vi "ex_getWaveformName.vi"(8 "error in (no error)":errorcluster, 10 "TimeColumnMode":T1, 11 "Dynamic Data":waveform(dbl)[](array[waveform])) -> (0 "error out":errorcluster, 3 "WaveName":string[](array[string]))   [LabVIEW 2017]
uses:
  <vilib>/express/express shared/NI_ExcelFile/Ctrls/TimeColumnMode.ctl
  <vilib>/express/express shared/NI_ExcelFile/NI_ExcelFile.lvlib
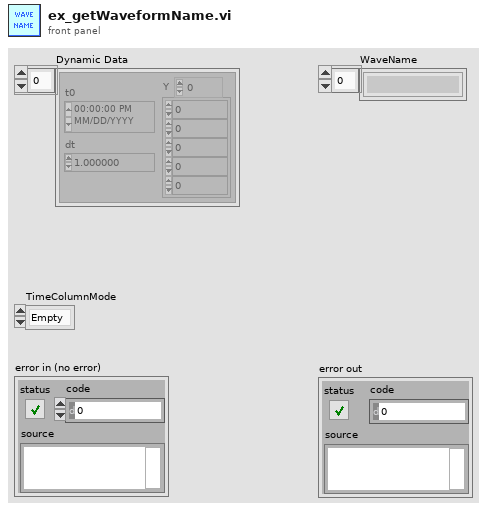
[diagram p1: front panel]
types:
  T1 = typedef "NI_ExcelFile.lvlib/TimeColumnMode.ctl" = enum16{"Empty", "OnePerCh", "One"}
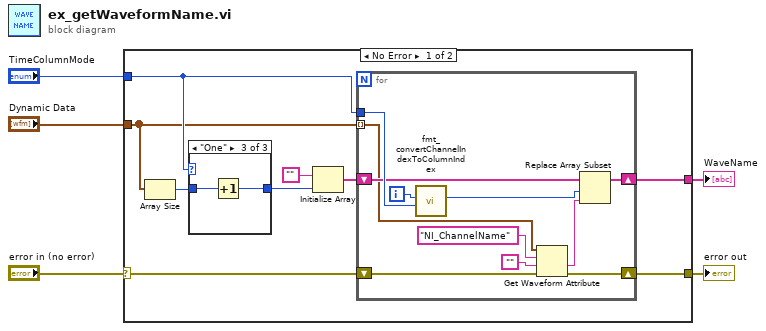
[diagram p0: block diagram]
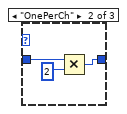
[diagram p3: hidden frame]
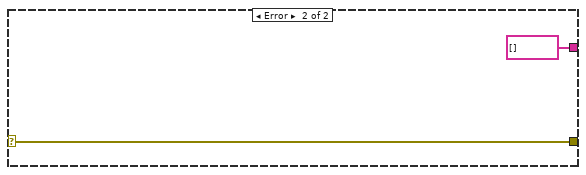
[diagram p4: hidden frame]
diagram:
  n1 = case shown="No Error" "error in (no error)" {
    selector: "error in (no error)" -> [w8 w33]
    tunnel: [w10 string[] []] -> w5
    tunnel: "Dynamic Data" -> [w7 _]
    tunnel: [w6 w33] -> w2
    tunnel: "TimeColumnMode" -> [w9 _]
    frame No Error {
      n2 = Array Size(array=w7) -> (size(s)=w13:i32)
      n3 = case shown="\"One\"" w9 {
        tunnel: w13 -> [w15 w18 w20]
        tunnel: [w15 w16 w19] -> w12
        frame "Empty", Default {
        }
        frame "OnePerCh" {
          n4 = Multiply(x=w18, y=2) -> (x*y=w16:i32)
        }
        frame "One" {
          n5 = Increment(x=w20) -> (x+1=w19:i32)
        }
      }
      n6 = Initialize Array("", w12) -> (w11:string[])
      n7 = for {
        tunnel: w9 -> [w29]
        shift-right: [w25] -> w10
        shift-left: w11 -> [w26]
        shift-right: [w23] -> w6
        shift-left: w8 -> [w24]
        tunnel: w7 -> [w22] mode=indexing
        i -> [w21]
        n8 = call <vilib>:"fmt_convertChannelIndexToColumnIndex.vi"("TimeColumnMode"=w29, "channel index"=w21) -> ("data column index"=w28:i32)  [unwired: 8 in, 1 out]
        n9 = Get Waveform Attribute(4:w24, 5:"", 6:"NI_ChannelName" ("name"), 7:w22) -> (0:w23:errorcluster, 1:w27:string)  [unwired: 2 out]
        n10 = Replace Array Subset(array=w26, new element=w27, index=w28) -> (w25:string[])
      }
    }
    frame Error {
    }
  }
  "error out" <- w2
  "WaveName" <- w5
